vi "AddTestMethod_Item_OnPopupMenu.vi"(11 "Object":T1) -> ()   [LabVIEW 2013]
uses:
  <resource>/Framework/Providers/API/ItemRef.ctl
  <resource>/Framework/Providers/API/mxLvMenuItem.ctl
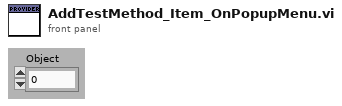
[diagram p1: front panel]
types:
  T1 = typedef "ItemRef.ctl" = u64
  T2 = typedef "mxLvMenuItem.ctl" = cluster{"Menu Name":string, "Description":string, "Icon File Name":path, "Menu Tag":string, "Enabled":bool, "Checked":bool, "Separator":bool, "Batchable":bool, "Weight":i32, "Batch Mode (Ignored if Not Batchable)":enum32{"Show If All Items Support Command", "Show If Any Items Support Command"}, "Menu Location":enum32{"<None>", "Project", "Project / Build Specifications", "Tools", "Tools / Source Control", "Tools / Real-Time Module", "Help"}, "Exclude From Getting Started Window Menu":bool}
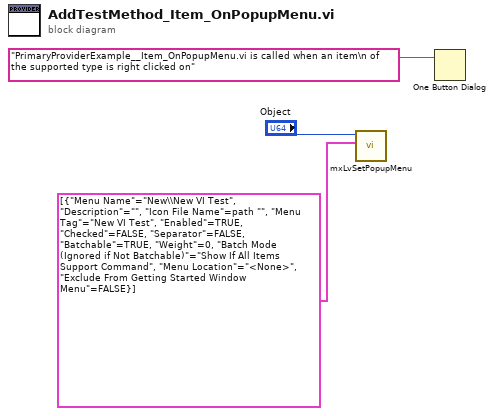
[diagram p0: block diagram]
diagram:
  n1 = call <resource>:"mxLvSetPopupMenu.vi"("Popup Menu Items"=T2[] [{"Menu Name"="New\\New VI Test", "Description"="", "Icon File Name"=path "", "Menu Tag"="New VI Test", "Enabled"=TRUE, "Checked"=FALSE, "Separator"=FALSE, "Batchable"=TRUE, "Weight"=0, "Batch Mode (Ignored if Not Batchable)"=enum."Show If All Items Support Command", "Menu Location"=enum."<None>", "Exclude From Getting Started Window Menu"=FALSE}], "Item"="Object") -> ()  [unwired: 8 in, 2 out]
  n2 = One Button Dialog(message="PrimaryProviderExample__Item_OnPopupMenu.vi is called when an item\n of the supported type is right clicked on") -> ()  [unwired: 1 in, 1 out]
